vi "continous-soliton-trigger-test.vi"() -> ()   [LabVIEW 2011]
doc: "This example demonstrates how to generate a single pulse using a counter output. \n\nThe single pulse may be triggered once or repeatedly from an external source."
uses:
  <vilib>/Utility/error.llb/DialogType.ctl
  <vilib>/DAQmx/create/channels.llb/DAQmx Create Channel (CO-Pulse Generation-Time).vi
  Program Files (x86)/National Instruments/LabVIEW 2011/resource/objmgr/daqmx.rc
panel:
  in  "milliseconds to trigger":u32=100
  in  "Continous trigger?":bool=TRUE
  in  "stop":bool
  out "number of trigger":i32=32
  in  "Stop":bool
  in  "Pulse Duration":dbl=0.0001 format="%.6f"
  in  "Output Terminal":tag="/Dev1/PFI0"
  in  "Counter":tag="Dev1/ctr0"
  # "Channel Settings"
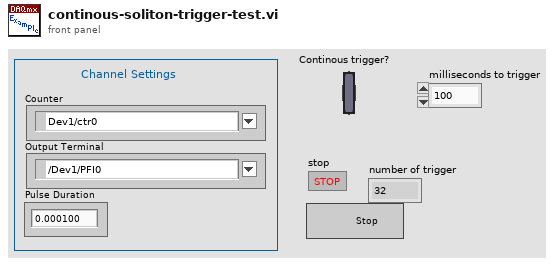
[diagram p1: front panel]
types:
  T1 = typedef "DialogType.ctl" = u16
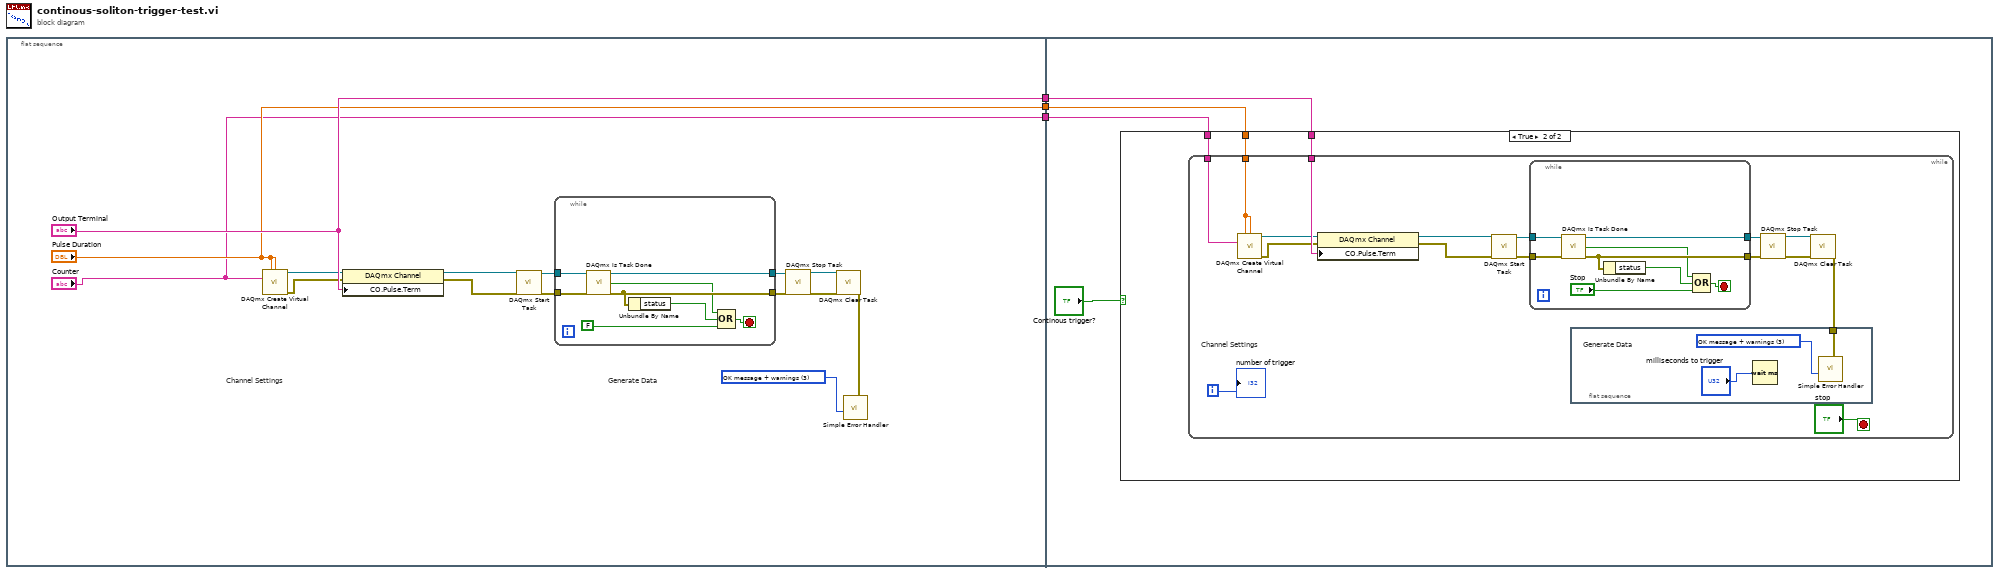
[diagram p0: block diagram]
diagram:
  n1 = flat-sequence {
    tunnel: ["Output Terminal"] -> w3
    tunnel: ["Pulse Duration"] -> w2
    tunnel: ["Counter"] -> w1
    tunnel: w3 -> [w27]
    tunnel: w2 -> [w28]
    tunnel: w1 -> [w29]
    frame #0 {
      w6 = T1 3 items=["no dialog", "OK message", "continue or stop message", "OK message + warnings", "continue/stop + warnings"] ("type of dialog (OK msg:1)")
      # "Generate Data"
      # "Channel Settings"
      n2 = call-poly <vilib>:"DAQmx Create Virtual Channel.vi"("high time"="Pulse Duration", "low time"="Pulse Duration", "counter"="Counter") -> ("task out"=w12:refnum<k21>, "error out"=w11:errorcluster)  [unwired: 11 in]
      n3 = property class="DAQmx Channel"(reference=w12, error in=w11, "CO.Pulse.Term"="Output Terminal") -> (reference out=w4:refnum<k21>, error out=w5:errorcluster)
      n4 = call <vilib>:"DAQmx Start Task.vi"("task/channels in"=w4, "error in"=w5) -> ("task out"=w15:refnum<k21>, "error out"=w14:errorcluster)  [unwired: 12 in]
      n5 = while {
        tunnel: w15 -> [w26]
        tunnel: w14 -> [w25]
        tunnel: [w22] -> w9
        tunnel: [w23] -> w10
        stop <- w24 stop-if-true
        n6 = call <vilib>:"DAQmx Is Task Done.vi"("task/channels in"=w26, "error in"=w25) -> ("task out"=w23:refnum<k21>, "task done?"=w19:bool, "error out"=w22:errorcluster)  [unwired: 11 in]
        n7 = Unbundle By Name(w22) -> ("status"=w21:bool)
        n8 = Compound Arithmetic op=OR(w19, w21, FALSE ("Stop 2")) -> (w24:bool)
      }
      n9 = call <vilib>:"DAQmx Stop Task.vi"("task/channels in"=w10, "error in"=w9) -> ("task out"=w8:refnum<k21>, "error out"=w7:errorcluster)  [unwired: 12 in]
      n10 = call <vilib>:"DAQmx Clear Task.vi"("task in"=w8, "error in"=w7) -> ("error out"=w13:errorcluster)  [unwired: 13 in]
      n11 = call <vilib>:"Simple Error Handler.vi"("type of dialog (OK msg:1)"=w6, "error in (no error)"=w13) -> ()  [unwired: 3 in, 5 out]
    }
    frame #1 {
      n12 = case shown="True" "Continous trigger?" {
        tunnel: w27 -> [_ w33]
        tunnel: w28 -> [_ w32]
        tunnel: w29 -> [_ w31]
        frame False {
        }
        frame True {
          n13 = while {
            tunnel: w33 -> [w47]
            tunnel: w32 -> [w46]
            tunnel: w31 -> [w45]
            i -> [w48]
            stop <- "stop" stop-if-true
            # "Channel Settings"
            n14 = call-poly <vilib>:"DAQmx Create Virtual Channel.vi"("high time"=w46, "low time"=w46, "counter"=w45) -> ("task out"=w41:refnum<k21>, "error out"=w40:errorcluster)  [unwired: 11 in]
            n15 = property class="DAQmx Channel"(reference=w41, error in=w40, "CO.Pulse.Term"=w47) -> (reference out=w34:refnum<k21>, error out=w35:errorcluster)
            n16 = call <vilib>:"DAQmx Start Task.vi"("task/channels in"=w34, "error in"=w35) -> ("task out"=w44:refnum<k21>, "error out"=w43:errorcluster)  [unwired: 12 in]
            n17 = while {
              tunnel: w44 -> [w60]
              tunnel: w43 -> [w59]
              tunnel: [w56] -> w38
              tunnel: [w57] -> w39
              stop <- w58 stop-if-true
              n18 = call <vilib>:"DAQmx Is Task Done.vi"("task/channels in"=w60, "error in"=w59) -> ("task out"=w57:refnum<k21>, "task done?"=w53:bool, "error out"=w56:errorcluster)  [unwired: 11 in]
              n19 = Unbundle By Name(w56) -> ("status"=w55:bool)
              n20 = Compound Arithmetic op=OR(w53, w55, "Stop") -> (w58:bool)
            }
            n21 = flat-sequence {
              tunnel: w42 -> [w52]
              frame #0 {
                w51 = T1 3 items=["no dialog", "OK message", "continue or stop message", "OK message + warnings", "continue/stop + warnings"] ("type of dialog (OK msg:1)")
                # "Generate Data"
                n22 = Wait (ms)(milliseconds to wait="milliseconds to trigger") -> ()  [unwired: 1 out]
                n23 = call <vilib>:"Simple Error Handler.vi"("type of dialog (OK msg:1)"=w51, "error in (no error)"=w52) -> ()  [unwired: 3 in, 5 out]
              }
            }
            n24 = call <vilib>:"DAQmx Stop Task.vi"("task/channels in"=w39, "error in"=w38) -> ("task out"=w37:refnum<k21>, "error out"=w36:errorcluster)  [unwired: 12 in]
            n25 = call <vilib>:"DAQmx Clear Task.vi"("task in"=w37, "error in"=w36) -> ("error out"=w42:errorcluster)  [unwired: 13 in]
            "number of trigger" <- w48
          }
        }
      }
    }
  }
